vi "Assert Result.vi"(8 "error in (no error)":errorcluster, 9 "Mock":refnum<class "Mock.lvclass">, 10 "Status":T1(ring), 11 "One Expectation Test In":refnum<class "One Expectation Test.lvclass">) -> (0 "error out":errorcluster, 3 "One Expectation Test Out":refnum<class "One Expectation Test.lvclass">)   [LabVIEW 2020, in "Expectation Test.lvclass"]
uses:
  Expectation Test/Expectation Test.lvclass
  One Expectation Test.lvclass
  C:/Program Files (x86)/National Instruments/LabVIEW 2020/vi.lib/Astemes/LUnit/Test Case.lvclass
  Mock/Mock.lvclass
  <vilib>/Astemes/LUnit/Test Case.lvclass
  <vilib>/Astemes/LUnit/Test Case.lvclass/Test Case.ctl
  c46993f4-e485-4ac3-9b25-20f97047735b.vi
  <vilib>/Astemes/LUnit/Append Pass Result.vi
  <vilib>/Astemes/LUnit/Append Fail Result.vi
  <vilib>/Astemes/LUnit/Describe Comparison.vi
  <vilib>/Astemes/LUnit/Compare Variants.vi
  <vilib>/Astemes/LUnit/Variant to string.vi
  <vilib>/Utility/Data Type/Get Type Information.vi
  <vilib>/Utility/LVClass/Get LV Class Name.vi
  Validator/Verifier.lvclass
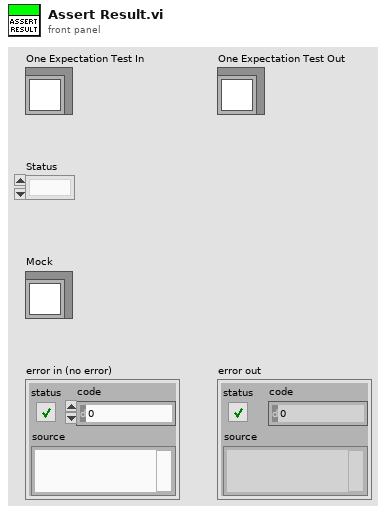
[diagram p1: front panel]
types:
  T1 = enum16{"", "Passed", "Failed", "Error", "Skipped", "Setup Error", "Broken", "Teardown Error"}
  T2 = cluster{"Name":string, "Message":string, "Description":string, "Status":enum16{"", "Passed", "Failed", "Error", "Skipped", "Setup Error", "Broken", "Teardown Error"}, "Result Type":enum16{"Test Case", "Test Suite", "Test Run", "Pass", "Fail", "Skip", "Pass if", "Fail if", "Pass if Error", "Fail if Error", "Pass if Equal", "Fail if Equal"}, "Execution Time":dbl}[]
  T3 = cluster{"Name":string, "Message":string, "Description":string, "Status":enum16{"", "Passed", "Failed", "Error", "Skipped", "Setup Error", "Broken", "Teardown Error"}, "Result Type":enum16{"Test Case", "Test Suite", "Test Run", "Pass", "Fail", "Skip", "Pass if", "Fail if", "Pass if Error", "Fail if Error", "Pass if Equal", "Fail if Equal"}, "Execution Time":dbl}
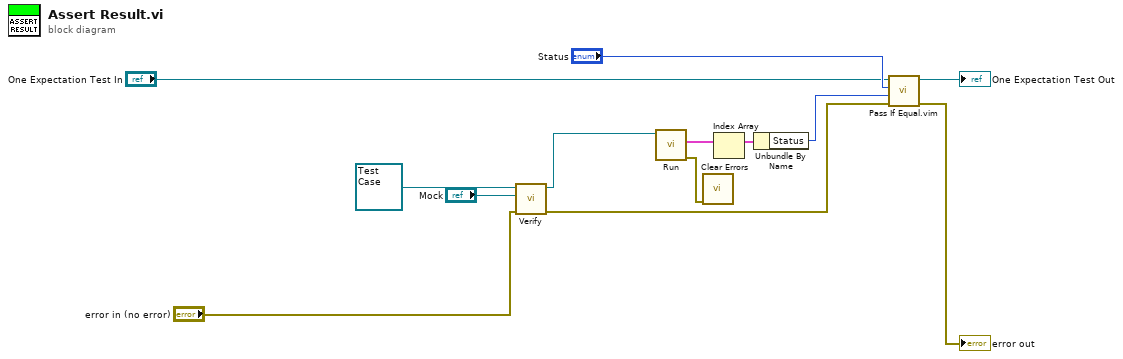
[diagram p0: block diagram]
diagram:
  n1 = call "Verify.vi"("error in (no error)"="error in (no error)", "Mock.lvclass"="Mock", "LUnit Test Case In"=refnum<class "Test Case.lvclass"> refnum) -> ("error out"=w1:errorcluster, "LUnit Test Case Out"=w4:refnum<class "Test Case.lvclass">)  [unwired: 7 in]
  n2 = call-dynamic "Run.vi"("LUnit Test Case In"=w4) -> ("error out"=w13:errorcluster, "Results"=w9:T2)  [unwired: 7 in, 2 out]
  n3 = call <vilib>:"Clear Errors.vi"("error in (no error)"=w13) -> ()  [unwired: 5 in, 2 out]
  n4 = Index Array(array=w9) -> (element=w10:T3)  [unwired: 1 in]
  n5 = Unbundle By Name(w10) -> ("Status"=w11:T1)
  n6 = call "Pass If Equal.vim"("error in (no error)"=w1, "Actual"=w11, "Expected"="Status", "LUnit Test Case In"="One Expectation Test In") -> ("error out"=→"error out":errorcluster, "LUnit Test Case Out"=→"One Expectation Test Out":refnum<class "One Expectation Test.lvclass">)  [unwired: 6 in]
